vi "WildDrive_v3.vi"(6 "Enter Pivot":bool, 10 "Turn Joystick":dbl, 11 "Speed Joystick":dbl=-0.0) -> (0 "Right Side Power":dbl, 3 "Left Side Power":dbl)   [LabVIEW 2018]
uses:
  <vilib>/Analysis/1siggen.llb/Ramp Pattern by Samples.vi
  <vilib>/Analysis/NI_AALBase.lvlib
panel:
  in  "Max Pivot Turn":dbl=0.35
  in  "Turn Behavior":bool=TRUE
  in  "Feed Forward":dbl=0.05
  in  "Debug Speed":dbl
  in  "Debug Mode":bool
  in  "Arc Turn Tuning":dbl=1.2
  out "Left Side Power":cluster{"Y":dbl[], "X":dbl[]}(graph)={"Y"=[0.0, 0.010101010101010102, 0.020202020202020204, 0.030303030303030304, 0.04040404040404041, 0.05050505050505051, 0.06060606060606061, 0.07070707070707072, 0.08080808080808081, 0.09090909090909091, 0.10101010101010102, 0.11111111111111112, 0.12121212121212122, 0.13131313131313133, 0.14141414141414144, 0.15151515151515152, 0.16161616161616163, 0.17171717171717174, 0.18181818181818182, 0.19191919191919193, 0.20202020202020204, 0.21212121212121213, 0.22222222222222224, 0.23232323232323235, 0.24242424242424243, 0.25252525252525254, 0.26262626262626265, 0.27272727272727276, 0.2828282828282829, 0.29292929292929293, 0.30303030303030304, 0.31313131313131315, 0.32323232323232326, 0.33333333333333337, 0.3434343434343435, 0.3535353535353536, 0.36363636363636365, 0.37373737373737376, 0.38383838383838387, 0.393939393939394, 0.4040404040404041, 0.4141414141414142, 0.42424242424242425, 0.43434343434343436, 0.4444444444444445, 0.4545454545454546, 0.4646464646464647, 0.4747474747474748, 0.48484848484848486, 0.494949494949495, 0.5050505050505051, 0.5151515151515152, 0.5252525252525253, 0.5353535353535354, 0.5454545454545455, 0.5555555555555556, 0.5656565656565657, 0.5757575757575758, 0.5858585858585859, 0.595959595959596, 0.6060606060606061, 0.6161616161616162, 0.6262626262626263, 0.6363636363636365, 0.6464646464646465, 0.6565656565656566, 0.6666666666666667, 0.6767676767676768, 0.686868686868687, 0.696969696969697, 0.7070707070707072, 0.7171717171717172, 0.7272727272727273, 0.7373737373737375, 0.7474747474747475, 0.7575757575757577, 0.7676767676767677, 0.7777777777777778, 0.787878787878788, 0.797979797979798, 0.8080808080808082, 0.8181818181818182, 0.8282828282828284, 0.8383838383838385, 0.8484848484848485, 0.8585858585858587, 0.8686868686868687, 0.8787878787878789, 0.888888888888889, 0.8989898989898991, 0.9090909090909092, 0.9191919191919192, 0.9292929292929294, 0.9393939393939394, 0.9494949494949496, 0.9595959595959597, 0.9696969696969697, 0.9797979797979799, 0.98989898989899, 1.0], "X"=[0.0]}
  out "Right Side Power":cluster{"Y":dbl[], "X":dbl[]}(graph)={"Y"=[0.0, 0.010101010101010102, 0.020202020202020204, 0.030303030303030304, 0.04040404040404041, 0.05050505050505051, 0.06060606060606061, 0.07070707070707072, 0.08080808080808081, 0.09090909090909091, 0.10101010101010102, 0.11111111111111112, 0.12121212121212122, 0.13131313131313133, 0.14141414141414144, 0.15151515151515152, 0.16161616161616163, 0.17171717171717174, 0.18181818181818182, 0.19191919191919193, 0.20202020202020204, 0.21212121212121213, 0.22222222222222224, 0.23232323232323235, 0.24242424242424243, 0.25252525252525254, 0.26262626262626265, 0.27272727272727276, 0.2828282828282829, 0.29292929292929293, 0.30303030303030304, 0.31313131313131315, 0.32323232323232326, 0.33333333333333337, 0.3434343434343435, 0.3535353535353536, 0.36363636363636365, 0.37373737373737376, 0.38383838383838387, 0.393939393939394, 0.4040404040404041, 0.4141414141414142, 0.42424242424242425, 0.43434343434343436, 0.4444444444444445, 0.4545454545454546, 0.4646464646464647, 0.4747474747474748, 0.48484848484848486, 0.494949494949495, 0.5050505050505051, 0.5151515151515152, 0.5252525252525253, 0.5353535353535354, 0.5454545454545455, 0.5555555555555556, 0.5656565656565657, 0.5757575757575758, 0.5858585858585859, 0.595959595959596, 0.6060606060606061, 0.6161616161616162, 0.6262626262626263, 0.6363636363636365, 0.6464646464646465, 0.6565656565656566, 0.6666666666666667, 0.6767676767676768, 0.686868686868687, 0.696969696969697, 0.7070707070707072, 0.7171717171717172, 0.7272727272727273, 0.7373737373737375, 0.7474747474747475, 0.7575757575757577, 0.7676767676767677, 0.7777777777777778, 0.787878787878788, 0.797979797979798, 0.8080808080808082, 0.8181818181818182, 0.8282828282828284, 0.8383838383838385, 0.8484848484848485, 0.8585858585858587, 0.8686868686868687, 0.8787878787878789, 0.888888888888889, 0.8989898989898991, 0.9090909090909092, 0.9191919191919192, 0.9292929292929294, 0.9393939393939394, 0.9494949494949496, 0.9595959595959597, 0.9696969696969697, 0.9797979797979799, 0.98989898989899, 1.0], "X"=[0.0]}
  in  "Turn Deadband":dbl=0.05 format="%#_13g"
  in  "Speed Deadband":dbl=0.05 format="%#_13g"
  out "Speed Joystick Mapping":cluster{"Y":dbl[], "X":dbl[]}(graph)={"Y"=[0.0, 0.010101010101010102, 0.020202020202020204, 0.030303030303030304, 0.04040404040404041, 0.05050505050505051, 0.06060606060606061, 0.07070707070707072, 0.08080808080808081, 0.09090909090909091, 0.10101010101010102, 0.11111111111111112, 0.12121212121212122, 0.13131313131313133, 0.14141414141414144, 0.15151515151515152, 0.16161616161616163, 0.17171717171717174, 0.18181818181818182, 0.19191919191919193, 0.20202020202020204, 0.21212121212121213, 0.22222222222222224, 0.23232323232323235, 0.24242424242424243, 0.25252525252525254, 0.26262626262626265, 0.27272727272727276, 0.2828282828282829, 0.29292929292929293, 0.30303030303030304, 0.31313131313131315, 0.32323232323232326, 0.33333333333333337, 0.3434343434343435, 0.3535353535353536, 0.36363636363636365, 0.37373737373737376, 0.38383838383838387, 0.393939393939394, 0.4040404040404041, 0.4141414141414142, 0.42424242424242425, 0.43434343434343436, 0.4444444444444445, 0.4545454545454546, 0.4646464646464647, 0.4747474747474748, 0.48484848484848486, 0.494949494949495, 0.5050505050505051, 0.5151515151515152, 0.5252525252525253, 0.5353535353535354, 0.5454545454545455, 0.5555555555555556, 0.5656565656565657, 0.5757575757575758, 0.5858585858585859, 0.595959595959596, 0.6060606060606061, 0.6161616161616162, 0.6262626262626263, 0.6363636363636365, 0.6464646464646465, 0.6565656565656566, 0.6666666666666667, 0.6767676767676768, 0.686868686868687, 0.696969696969697, 0.7070707070707072, 0.7171717171717172, 0.7272727272727273, 0.7373737373737375, 0.7474747474747475, 0.7575757575757577, 0.7676767676767677, 0.7777777777777778, 0.787878787878788, 0.797979797979798, 0.8080808080808082, 0.8181818181818182, 0.8282828282828284, 0.8383838383838385, 0.8484848484848485, 0.8585858585858587, 0.8686868686868687, 0.8787878787878789, 0.888888888888889, 0.8989898989898991, 0.9090909090909092, 0.9191919191919192, 0.9292929292929294, 0.9393939393939394, 0.9494949494949496, 0.9595959595959597, 0.9696969696969697, 0.9797979797979799, 0.98989898989899, 1.0], "X"=[0.0]}
  in  "Squared":bool=TRUE
  out "Turn Joystick Mapping":cluster{"Y":dbl[], "X":dbl[]}(graph)={"Y"=[0.0, 0.010101010101010102, 0.020202020202020204, 0.030303030303030304, 0.04040404040404041, 0.05050505050505051, 0.06060606060606061, 0.07070707070707072, 0.08080808080808081, 0.09090909090909091, 0.10101010101010102, 0.11111111111111112, 0.12121212121212122, 0.13131313131313133, 0.14141414141414144, 0.15151515151515152, 0.16161616161616163, 0.17171717171717174, 0.18181818181818182, 0.19191919191919193, 0.20202020202020204, 0.21212121212121213, 0.22222222222222224, 0.23232323232323235, 0.24242424242424243, 0.25252525252525254, 0.26262626262626265, 0.27272727272727276, 0.2828282828282829, 0.29292929292929293, 0.30303030303030304, 0.31313131313131315, 0.32323232323232326, 0.33333333333333337, 0.3434343434343435, 0.3535353535353536, 0.36363636363636365, 0.37373737373737376, 0.38383838383838387, 0.393939393939394, 0.4040404040404041, 0.4141414141414142, 0.42424242424242425, 0.43434343434343436, 0.4444444444444445, 0.4545454545454546, 0.4646464646464647, 0.4747474747474748, 0.48484848484848486, 0.494949494949495, 0.5050505050505051, 0.5151515151515152, 0.5252525252525253, 0.5353535353535354, 0.5454545454545455, 0.5555555555555556, 0.5656565656565657, 0.5757575757575758, 0.5858585858585859, 0.595959595959596, 0.6060606060606061, 0.6161616161616162, 0.6262626262626263, 0.6363636363636365, 0.6464646464646465, 0.6565656565656566, 0.6666666666666667, 0.6767676767676768, 0.686868686868687, 0.696969696969697, 0.7070707070707072, 0.7171717171717172, 0.7272727272727273, 0.7373737373737375, 0.7474747474747475, 0.7575757575757577, 0.7676767676767677, 0.7777777777777778, 0.787878787878788, 0.797979797979798, 0.8080808080808082, 0.8181818181818182, 0.8282828282828284, 0.8383838383838385, 0.8484848484848485, 0.8585858585858587, 0.8686868686868687, 0.8787878787878789, 0.888888888888889, 0.8989898989898991, 0.9090909090909092, 0.9191919191919192, 0.9292929292929294, 0.9393939393939394, 0.9494949494949496, 0.9595959595959597, 0.9696969696969697, 0.9797979797979799, 0.98989898989899, 1.0], "X"=[-0.0]}
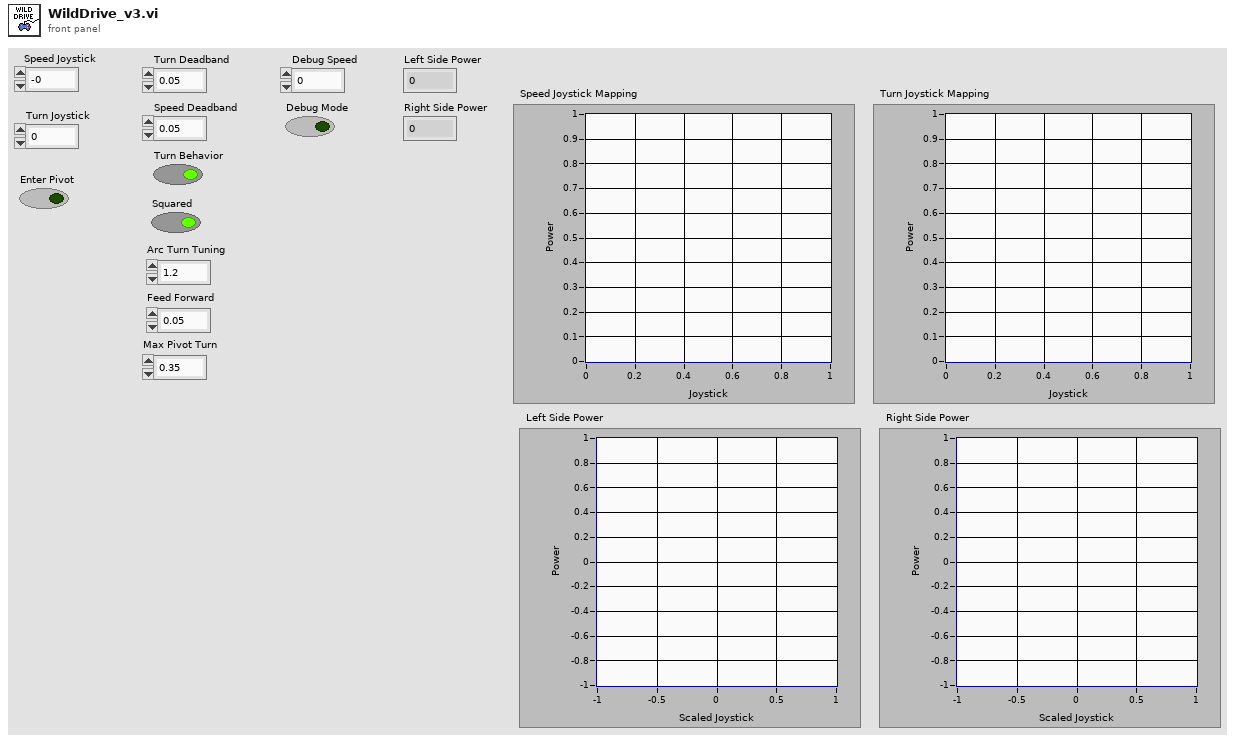
[diagram p1: front panel]
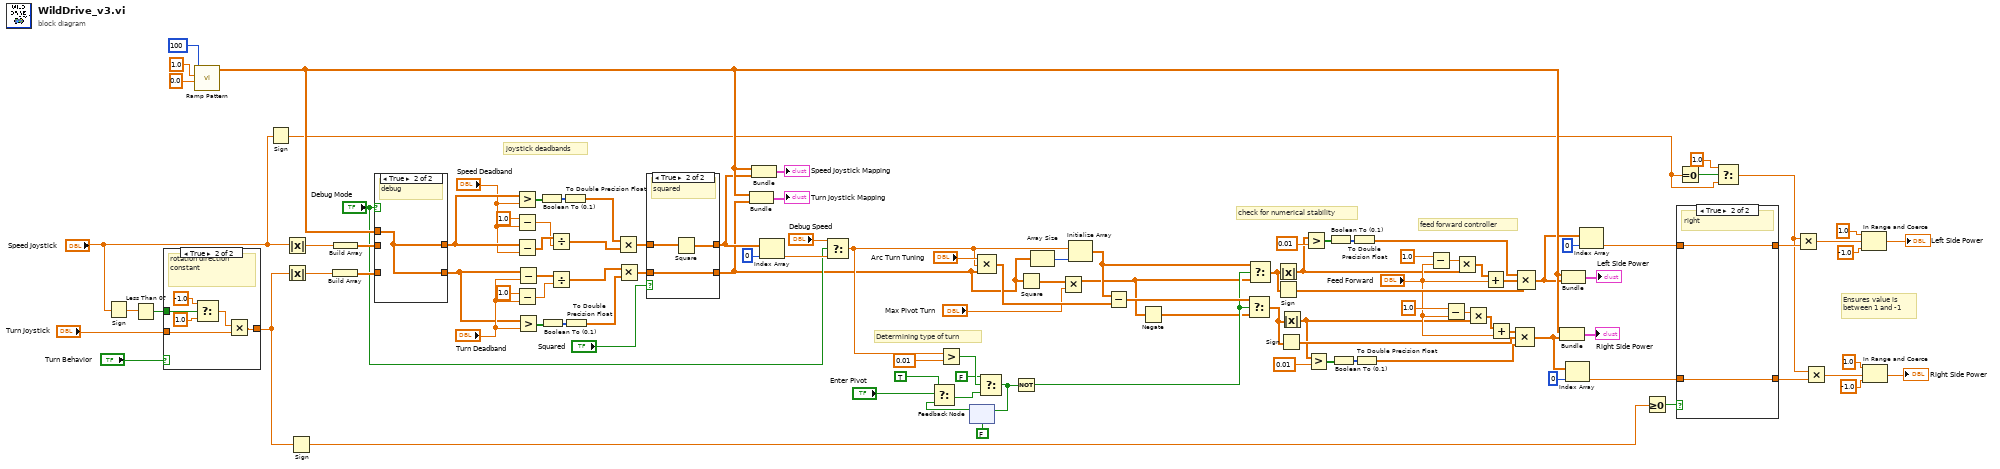
[diagram p0: block diagram]
diagram:
  # "check for numerical stability"
  # "Ensures value is \nbetween 1 and -1"
  # "Determining type of turn"
  # "feed forward controller"
  # "joystick deadbands"
  n1 = Sign(1:"Speed Joystick") -> (0:w12:dbl)
  n2 = Less Than 0?(x=w12) -> (x < 0?=w13:bool)
  n3 = case shown="True" "Turn Behavior" {
    tunnel: w13 -> [_ w116]
    tunnel: [w111 w113] -> w8
    tunnel: "Turn Joystick" -> [w111 w112]
    frame False {
      # "like a car"
    }
    frame True {
      # "rotation direction constant"
      n4 = Select(t=-1.0, s=w116, f=1.0) -> (s? t:f=w117:dbl)
      n5 = Multiply(x=w117, y=w112) -> (x*y=w113:dbl)
    }
  }
  n6 = call-poly <vilib>:"Ramp Pattern.vi"("start"=0.0, "end"=1.0, "samples"=100) -> ("Ramp Pattern"=w107:dbl[])  [unwired: 7 in, 1 out]
  n7 = Sign(1:"Speed Joystick") -> (0:w5:dbl)
  n8 = Absolute Value(x="Speed Joystick") -> (abs(x)=w102:dbl)
  n9 = Absolute Value(x=w8) -> (abs(x)=w105:dbl)
  n10 = Sign(1:w8) -> (0:w19:dbl)
  n11 = Build Array(w105) -> (w103:dbl[])
  n12 = Build Array(w102) -> (w104:dbl[])
  n13 = case shown="True" "Debug Mode" {
    tunnel: w107 -> [_ w120]
    tunnel: [w119 w120] -> w92
    tunnel: [w118 w120] -> w83
    tunnel: w104 -> [w119 _]
    tunnel: w103 -> [w118 _]
    frame False {
      # "normal"
    }
    frame True {
      # "debug"
    }
  }
  n14 = Greater?(x=w92, y="Speed Deadband") -> (0:w99:bool[])
  n15 = Subtract(x=1.0, y="Speed Deadband") -> (x-y=w89:dbl)
  n16 = Subtract(x=w92, y="Speed Deadband") -> (x-y=w91:dbl[])
  n17 = Subtract(x=1.0, y="Turn Deadband") -> (x-y=w85:dbl)
  n18 = Subtract(x=w83, y="Turn Deadband") -> (x-y=w87:dbl[])
  n19 = Greater?(x=w83, y="Turn Deadband") -> (0:w97:bool[])
  n20 = Boolean To (0,1)(Boolean=w99) -> (0, 1=w98:i16[])
  n21 = Boolean To (0,1)(Boolean=w97) -> (0, 1=w96:i16[])
  n22 = Divide(x=w91, y=w89) -> (x/y=w88:dbl[])
  n23 = Divide(x=w87, y=w85) -> (x/y=w82:dbl[])
  n24 = To Double Precision Float(number=w98) -> (double precision float=w94:dbl[])
  n25 = To Double Precision Float(number=w96) -> (double precision float=w81:dbl[])
  n26 = Multiply(x=w94, y=w88) -> (x*y=w93:dbl[])
  n27 = Multiply(x=w82, y=w81) -> (x*y=w95:dbl[])
  n28 = case shown="True" "Squared" {
    tunnel: w93 -> [w122 w125]
    tunnel: w95 -> [w121 w123]
    tunnel: [w122 w124] -> w66
    tunnel: [w121 w123] -> w17
    frame False {
      # "linear"
    }
    frame True {
      # "squared"
      n29 = Square(x=w125) -> (x^2=w124:dbl[])
    }
  }
  n30 = Bundle("Ramp Pattern"=w107, w17) -> (→"Turn Joystick Mapping":cluster{"Ramp Pattern":dbl[], dbl[]})  [unwired: 1 in]
  n31 = Bundle("Ramp Pattern"=w107, w66) -> (→"Speed Joystick Mapping":cluster{"Ramp Pattern":dbl[], dbl[]})  [unwired: 1 in]
  n32 = Index Array(array=w66, index=0) -> (element=w68:dbl)
  n33 = Select(t="Debug Speed", s="Debug Mode", f=w68) -> (s? t:f=w18:dbl)
  n34 = Greater?(x=w18, y=0.01) -> (0:w62:bool)
  n35 = feedback #1(FALSE) -> (w71:bool)
  n36 = Select(t=TRUE, s="Enter Pivot", f=w71) -> (s? t:f=w61:bool)
  n37 = Compound Arithmetic op=MULTIPLY("Arc Turn Tuning", w18, w17) -> (w73:dbl[])
  n38 = Select(t=FALSE, s=w62, f=w61) -> (s? t:f=w59:bool)
  n39 = feedback-in #1(w59) -> ()
  n40 = Not(x=w59) -> (.not. x?=w58:bool)
  n41 = Square(x=w17) -> (x^2=w3:dbl[])
  n42 = Array Size(array=w17) -> (size(s)=w79:i32)
  n43 = Multiply(x=w3, y="Max Pivot Turn") -> (x*y=w2:dbl[])
  n44 = Initialize Array(w18, w79) -> (w78:dbl[])
  n45 = Subtract(x=w78, y=w73) -> (x-y=w77:dbl[])
  n46 = Negate(x=w2) -> (-x=w57:dbl[])
  n47 = Select(t=w77, s=w58, f=w57) -> (s? t:f=w16:dbl[])
  n48 = Select(t=w78, s=w58, f=w2) -> (s? t:f=w39:dbl[])
  n49 = Sign(1:w39) -> (0:w53:dbl[])
  n50 = Absolute Value(x=w39) -> (abs(x)=w14:dbl[])
  n51 = Sign(1:w16) -> (0:w48:dbl[])
  n52 = Absolute Value(x=w16) -> (abs(x)=w15:dbl[])
  n53 = Greater?(x=w14, y=0.01) -> (0:w42:bool[])
  n54 = Greater?(x=w15, y=0.01) -> (0:w46:bool[])
  n55 = Boolean To (0,1)(Boolean=w42) -> (0, 1=w41:i16[])
  n56 = Boolean To (0,1)(Boolean=w46) -> (0, 1=w45:i16[])
  n57 = To Double Precision Float(number=w41) -> (double precision float=w38:dbl[])
  n58 = To Double Precision Float(number=w45) -> (double precision float=w43:dbl[])
  n59 = Subtract(x=1.0, y="Feed Forward") -> (x-y=w55:dbl)
  n60 = Subtract(x=1.0, y="Feed Forward") -> (x-y=w51:dbl)
  n61 = Multiply(x=w55, y=w14) -> (x*y=w54:dbl[])
  n62 = Multiply(x=w51, y=w15) -> (x*y=w50:dbl[])
  n63 = Add(x=w54, y="Feed Forward") -> (x+y=w37:dbl[])
  n64 = Add(x=w50, y="Feed Forward") -> (x+y=w49:dbl[])
  n65 = Compound Arithmetic op=MULTIPLY(w49, w48, w43) -> (w35:dbl[])
  n66 = Compound Arithmetic op=MULTIPLY(w38, w37, w53) -> (w33:dbl[])
  n67 = Bundle("Ramp Pattern"=w107, w35) -> (→"Right Side Power":cluster{"Ramp Pattern":dbl[], dbl[]})  [unwired: 1 in]
  n68 = Bundle("Ramp Pattern"=w107, w33) -> (→"Left Side Power":cluster{"Ramp Pattern":dbl[], dbl[]})  [unwired: 1 in]
  n69 = Index Array(array=w35, index=0) -> (element=w22:dbl)
  n70 = Index Array(array=w33, index=0) -> (element=w24:dbl)
  n71 = Greater Or Equal To 0?(x=w19) -> (x >= 0?=w20:bool)
  n72 = case shown="True" w20 {
    tunnel: w24 -> [w127 w129]
    tunnel: [w126 w129] -> w23
    tunnel: w22 -> [w126 w128]
    tunnel: [w127 w128] -> w21
    frame False {
      # "left"
    }
    frame True {
      # "right"
    }
  }
  n73 = Equal To 0?(x=w5) -> (x = 0?=w7:bool)
  n74 = Select(t=1.0, s=w7, f=w5) -> (s? t:f=w4:dbl)
  n75 = Multiply(x=w4, y=w23) -> (x*y=w25:dbl)
  n76 = Multiply(x=w4, y=w21) -> (x*y=w26:dbl)
  n77 = In Range and Coerce(upper limit=1.0, x=w25, lower limit=-1.0) -> (coerced(x)=→"Left Side Power":dbl)  [unwired: 1 out]
  n78 = In Range and Coerce(upper limit=1.0, x=w26, lower limit=-1.0) -> (coerced(x)=→"Right Side Power":dbl)  [unwired: 1 out]
